vi "Parse Nest Data.vi"() -> ()   [LabVIEW 2013, in "LMH-Nest.lvlib"]
uses:
  LMH-Nest.lvlib
  Type Defs/Nest Config.ctl
  <vilib>/httpClient/ClientHandle.ctl
  Type Defs/Session Data.ctl
  <vilib>/httpClient/LabVIEWHTTPClient.lvlib
panel:
  in  "Token":string="name"
  out "Device Name":string
  in  "Device ID":string
  out "Data":string
  out "Error Out":errorcluster
  in  "Error In":errorcluster
  out "Nest Config":T1
  in  "Nest Config":T1
  in  "Data":string
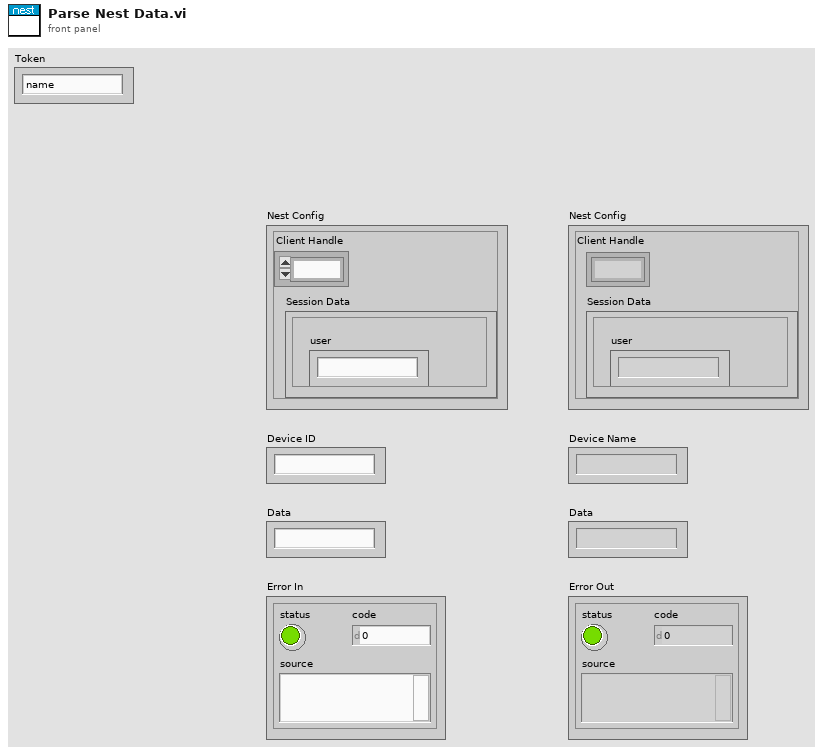
[diagram p1: front panel]
types:
  T1 = typedef "LMH-Nest.lvlib/Nest Config.ctl" = cluster{"Client Handle":T2, "Session Data":T3}
  T2 = typedef "LabVIEWHTTPClient.lvlib/ClientHandle.ctl" = refnum<k1>
  T3 = typedef "LMH-Nest.lvlib/Session Data.ctl" = cluster{"is_superuser":bool, "is_staff":bool, "urls":cluster{"transport_url":string, "rubyapi_url":string, "weather_url":string, "log_upload_url":string, "support_url":string}, "limits":cluster{"thermostats_per_structure":u32, "structures":u32, "thermostats":u32, "smoke_detectors":u32, "smoke_detectors_per_structure":u32}, "access_token":string, "userid":string, "expires_in":string, "email":string, "user":string, "language":string}
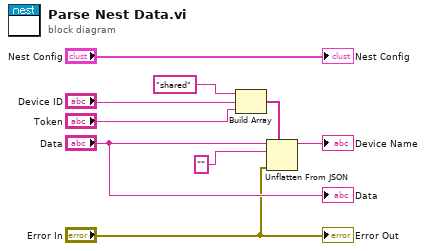
[diagram p0: block diagram]
diagram:
  n1 = Build Array("shared", "Device ID", "Token") -> (w5:string[])
  n2 = Unflatten From JSON(path=w5, JSON string="Data", type and defaults="", error in (no error)="Error In") -> (value=→"Device Name":string)  [unwired: 3 in, 1 out]
  "Nest Config" <- "Nest Config"
  "Error Out" <- "Error In"
  "Data" <- "Data"
